vi "Event Handle Loop_Set Active Button.vi"(8 "error in (no error)":errorcluster, 10 "Label":string, 11 "QMenu Class in":refnum<class "QMenu Class.lvclass">) -> (0 "error out":errorcluster, 3 "QMenu Class out":refnum<class "QMenu Class.lvclass">)   [LabVIEW 2020, in "QTab.lvlib" / "QMenu Class.lvclass"]
uses:
  QMenu Class.lvclass
  QMenu Class.lvclass/QMenu Class.ctl
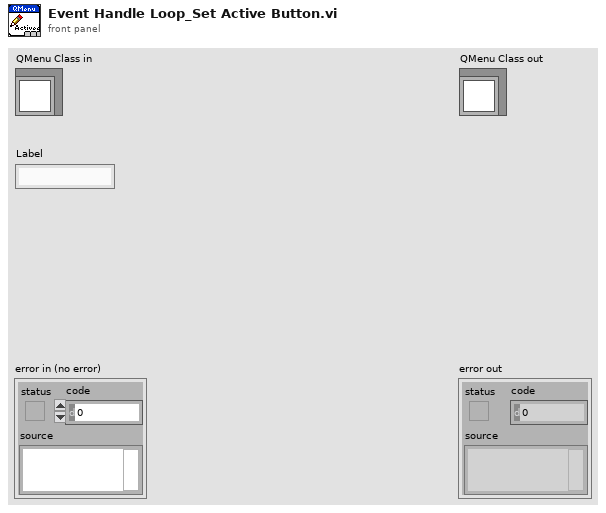
[diagram p1: front panel]
types:
  T1 = typedef "QTab.lvlib/QMenu Class.lvclass/Button Attribute.ctl" = cluster{"Label":string, "Button Text":string, "Closable":bool, "Draggable":bool}
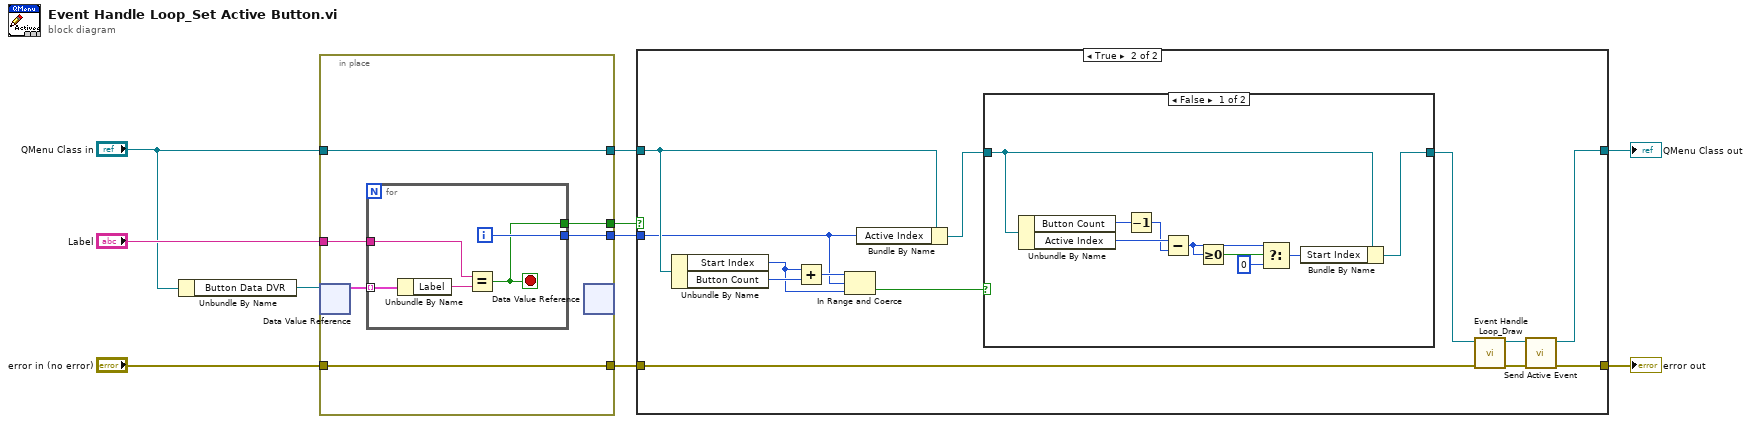
[diagram p0: block diagram]
diagram:
  n1 = Unbundle By Name("QMenu Class in") -> ("Button Data DVR"=w9:refnum<data-value>)
  n2 = in-place {
    in-place-border: "error in (no error)" -> [w11]
    in-place-border: "Label" -> [w14]
    in-place-border: "QMenu Class in" -> [w16]
    in-place-border: [w16] -> w3
    in-place-border: [w13] -> w4
    in-place-border: [w12] -> w5
    in-place-border: [w11] -> w6
    n3 = in-place-dvr #1(w9) -> (w15:T1[])  [unwired: 1 out]
    n4 = for {
      tunnel: w15 -> [w21] mode=indexing
      tunnel: w14 -> [w19]
      tunnel: [w18] -> w12
      tunnel: [w17] -> w13
      i -> [w18]
      stop <- w17 stop-if-true
      n5 = Unbundle By Name(w21) -> ("Label"=w20:string)
      n6 = Equal?(x=w19, y=w20) -> (x = y?=w17:bool)
    }
    n7 = in-place-dvr #1() -> ()  [unwired: 1 in, 2 out]
  }
  n8 = case shown="True" w4 {
    tunnel: [w23 w32] -> w1
    tunnel: [w22 w33] -> w2
    tunnel: w3 -> [w23 w27]
    tunnel: w6 -> [w22 w36]
    tunnel: w5 -> [_ w26]
    frame False {
    }
    frame True {
      n9 = Unbundle By Name(w27) -> ("Start Index"=w29:i32, "Button Count"=w31:i32)
      n10 = Add(x=w29, y=w31) -> (x+y=w30:i32)
      n11 = In Range and Coerce(upper limit=w30, x=w26, lower limit=w29) -> (In Range?=w28:bool)  [unwired: 1 out]
      n12 = Bundle By Name(cluster=w27, "Active Index"=w26) -> (w25:refnum<class "QMenu Class.lvclass">)
      n13 = case shown="False" w28 {
        tunnel: w25 -> [w45 w46]
        tunnel: [w44 w46] -> w24
        frame False {
          n14 = Unbundle By Name(w45) -> ("Button Count"=w42:i32, "Active Index"=w43:i32)
          n15 = Decrement(x=w42) -> (x-1=w41:i32)
          n16 = Subtract(x=w43, y=w41) -> (x-y=w39:i32)
          n17 = Greater Or Equal To 0?(x=w39) -> (x >= 0?=w40:bool)
          n18 = Select(t=w39, s=w40, f=0) -> (s? t:f=w37:i32)
          n19 = Bundle By Name(cluster=w45, "Start Index"=w37) -> (w44:refnum<class "QMenu Class.lvclass">)
        }
        frame True {
        }
      }
      n20 = call "Event Handle Loop_Draw.vi"("error in (no error)"=w36, "QMenu Class in"=w24) -> ("error out"=w35:errorcluster, "QMenu Class out"=w34:refnum<class "QMenu Class.lvclass">)  [unwired: 8 in]
      n21 = call "Send Active Event.vi"("error in (no error)"=w35, "QMenu Class in"=w34) -> ("error out"=w33:errorcluster, "QMenu Class out"=w32:refnum<class "QMenu Class.lvclass">)  [unwired: 8 in]
    }
  }
  "error out" <- w2
  "QMenu Class out" <- w1
